vi "Initialize Values.vi"(8 "error in (no error)":errorcluster, 11 "Measurement wRelev in":refnum<class "Measurement wRelev.lvclass">) -> (0 "error out":errorcluster, 3 "Measurement wRelev out":refnum<class "Measurement wRelev.lvclass">)   [LabVIEW 2014, in "SeqLoop.lvlib" / "STEP Classes.lvlib" / "Measurement wRelev.lvclass"]
uses:
  Measurement wRelev.lvclass
  Measurement wRelev.lvclass/Measurement wRelev.ctl
  STEP/STEP.lvclass
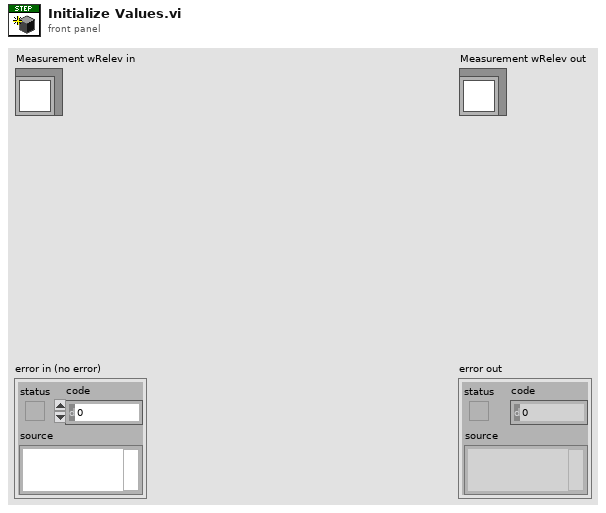
[diagram p1: front panel]
types:
  T1 = cluster{"HWAsync 1":string, "HWAsync 2":string, "HWAsync 3":string, "HWAsync 4":string, "HWAsync 5":string, "HWAsync 6":string, "HWAsync 7":string, "HWAsync 8":string, "HWAsync 9":string, "HWAsync 10":string}
  T2 = cluster{"HWSync 1":bool, "HWSync 2":bool, "HWSync 3":bool, "HWSync 4":bool, "HWSync 5":bool}
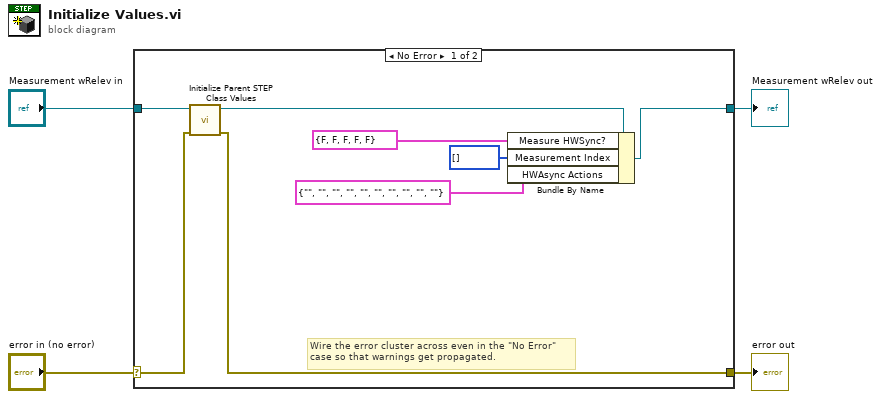
[diagram p0: block diagram]
diagram:
  n1 = case shown="No Error" "error in (no error)" {
    selector: "error in (no error)" -> [w12 w14]
    tunnel: [w11 w14] -> w3
    tunnel: [w8 w13] -> w1
    tunnel: "Measurement wRelev in" -> [w10 w13]
    frame No Error {
      # "Wire the error cluster across even in the \"No Error\"\ncase so that warnings get propagated."
      n2 = call "Initialize Parent STEP Class Values.vi"("error in (no error)"=w12, "STEP in"=w10) -> ("error out"=w11:errorcluster, "STEP out"=w9:refnum<class "Measurement wRelev.lvclass">)  [unwired: 8 in]
      n3 = Bundle By Name(cluster=w9, "Measure HWSync?"=T2 {"HWSync 1"=FALSE, "HWSync 2"=FALSE, "HWSync 3"=FALSE, "HWSync 4"=FALSE, "HWSync 5"=FALSE}, "Measurement Index"=i32[] [], "HWAsync Actions"=T1 {"HWAsync 1"="", "HWAsync 2"="", "HWAsync 3"="", "HWAsync 4"="", "HWAsync 5"="", "HWAsync 6"="", "HWAsync 7"="", "HWAsync 8"="", "HWAsync 9"="", "HWAsync 10"=""}) -> (w8:refnum<class "Measurement wRelev.lvclass">)
    }
    frame Error {
    }
  }
  "error out" <- w3
  "Measurement wRelev out" <- w1
